vi "Launch Event Handlers.vi"(8 "error in (no error)":errorcluster, 11 "IEventAggregator In":refnum<class "IEventAggregator.lvclass">) -> (0 "error out":errorcluster, 3 "IEventAggregator Out":refnum<class "IEventAggregator.lvclass">)   [LabVIEW 2015, in "ActorEvents.lvlib" / "IEventAggregator.lvclass"]
uses:
  IEventAggregator.lvclass
  IEventAggregator.lvclass/IEventAggregator.ctl
  IEventHandler/IEventHandler.lvclass
  <vilib>/ActorFramework/Actor/Actor.lvclass/Actor.ctl
  <vilib>/ActorFramework/Message Enqueuer/Message Enqueuer.lvclass/Message Enqueuer.ctl
  IEventHandler/IEventHandler.lvclass/IEventHandler.ctl
  <vilib>/ActorFramework/Actor/Read Self Enqueuer.vi
  <vilib>/ActorFramework/Message Enqueuer/Init from Existing Queue.vi
  <vilib>/ActorFramework/Actor/Launch Nested Actor.vi
  <vilib>/ActorFramework/Message Enqueuer/Message Enqueuer.lvclass
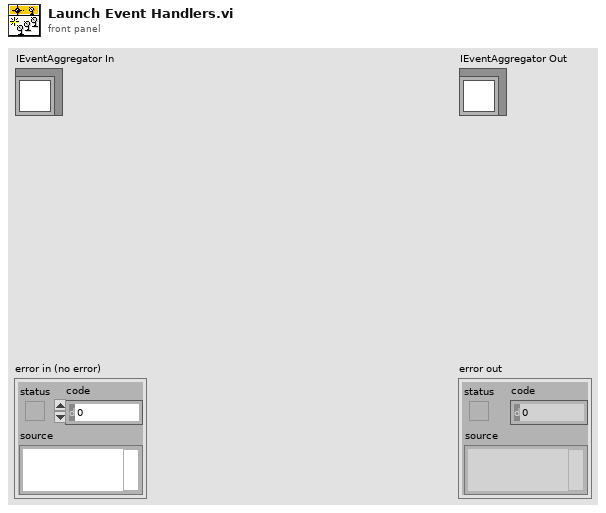
[diagram p1: front panel]
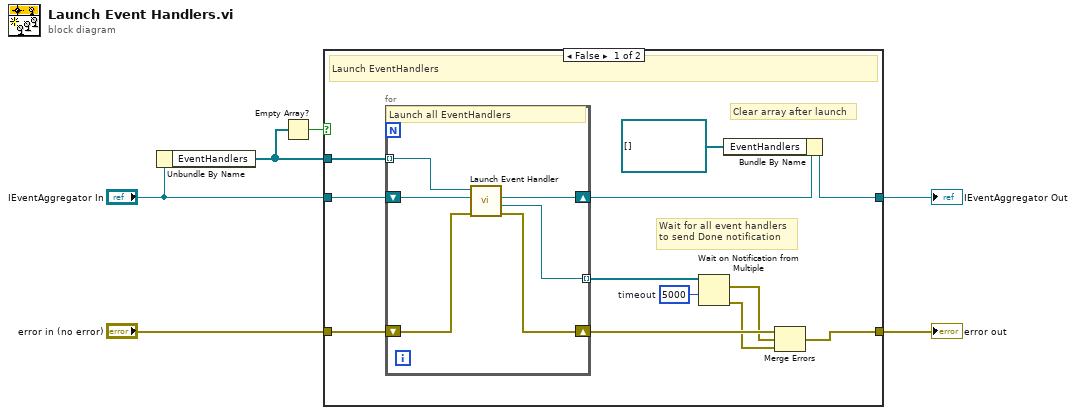
[diagram p0: block diagram]
diagram:
  n1 = Unbundle By Name("IEventAggregator In") -> ("EventHandlers"=w1:refnum<class "IEventHandler.lvclass">[])
  n2 = Empty Array?(array=w1) -> (empty?=w2:bool)
  n3 = case shown="False" w2 {
    tunnel: "error in (no error)" -> [w16 w25]
    tunnel: [w13 w25] -> w5
    tunnel: "IEventAggregator In" -> [w10 w26]
    tunnel: w1 -> [w9 _]
    tunnel: [w8 w26] -> w3
    frame False {
      w14 = 5000  # timeout
      # "Clear array after launch"
      # "Wait for all event handlers\nto send Done notification"
      # "Launch EventHandlers"
      n4 = for {
        shift-right: [w23] -> w18
        shift-left: w10 -> [w24]
        tunnel: w9 -> [w22] mode=indexing
        tunnel: [w21] -> w17 mode=indexing
        shift-right: [w20] -> w15
        shift-left: w16 -> [w19]
        # "Launch all EventHandlers"
        n5 = call "Launch Event Handler.vi"("error in (no error)"=w19, "EventAggregator In"=w24, "EventHandler In"=w22) -> ("error out"=w20:errorcluster, "Registration Done Notifier"=w21:refnum<notifier>, "EventAggregator Out"=w23:refnum<class "IEventAggregator.lvclass">)  [unwired: 5 in, 1 out]
      }
      n6 = Wait on Notification from Multiple(0:w17, 2:w14) -> (9:w12:errorcluster[], 11:w11:errorcluster)  [unwired: 2 in, 2 out]
      n7 = Bundle By Name(cluster=w18, "EventHandlers"=refnum<class "IEventHandler.lvclass">[] []) -> (w8:refnum<class "IEventAggregator.lvclass">)
      n8 = Merge Errors(w15, w12, w11) -> (w13:errorcluster)
    }
    frame True {
      # "Empty array -- No handlers to launch"
    }
  }
  "error out" <- w5
  "IEventAggregator Out" <- w3
